vi "Basic_SetupBoard.vi"() -> ()   [LabVIEW 2020]
uses:
  controls/basic_tx_states.ctl
  AIM664LV.lvlib
panel:
  in  "Explicit libInit (T)":bool=TRUE
  out "BSP Version Out":T1
  out "Board Control Out":T2 {"SharedMemFree" format="%x"; "GlobalMemFree" format="%x"; "ExpertMode" items=["FDX_EXPERT_MODE", "FDX_DISA_GHOST"]; "PortGoodLink" items=["FDX_NO_LINK", "FDX_GOOD_LINK"]; "PortSpeed" items=["FDX_100MBIT", "FDX_10MBIT", "FDX_AUTO_100MBIT", "FDX_AUTO_10MBIT", "FDX_AUTO_ERROR", "FDX_1000MBIT"]; "PortConfig" items=["FDX_SINGLE", "FDX_REDUNDANT"]}
  in  "ExpertMode":u32(ring) items=["FDX_EXPERT_MODE", "FDX_DISA_GHOST"]
  in  "PortSpeedIn":u32(ring) items=["FDX_100MBIT"=0, "FDX_10MBIT"=1, "FDX_AUTO_100MBIT"=2, "FDX_AUTO_10MBIT"=3, "FDX_1000MBIT"=5]
  in  "PortConfigIn":u32(ring) items=["FDX_SINGLE", "FDX_REDUNDANT"]
  in  "Control":u32(ring) items=["FDX_READ", "FDX_WRITE"]
  out "error out":errorcluster
  out "ServerResourceInfo":T3(array[cluster]) {"ResourceType" items=["RESOURCETYPE_BOARD"=0, "RESOURCETYPE_PORT"=1, "RESOURCETYPE_ALL"=20]}
  out "NuOfServers":u32
  # "#define FDX_100MBIT        0\n#define FDX_10MBIT         1\n#define FDX_AUTO_100MBIT   2\n#define FDX_AUTO_10MBIT    3\n#define FDX_AUTO_ERROR     4\n#define FDX_1000MBIT       5"
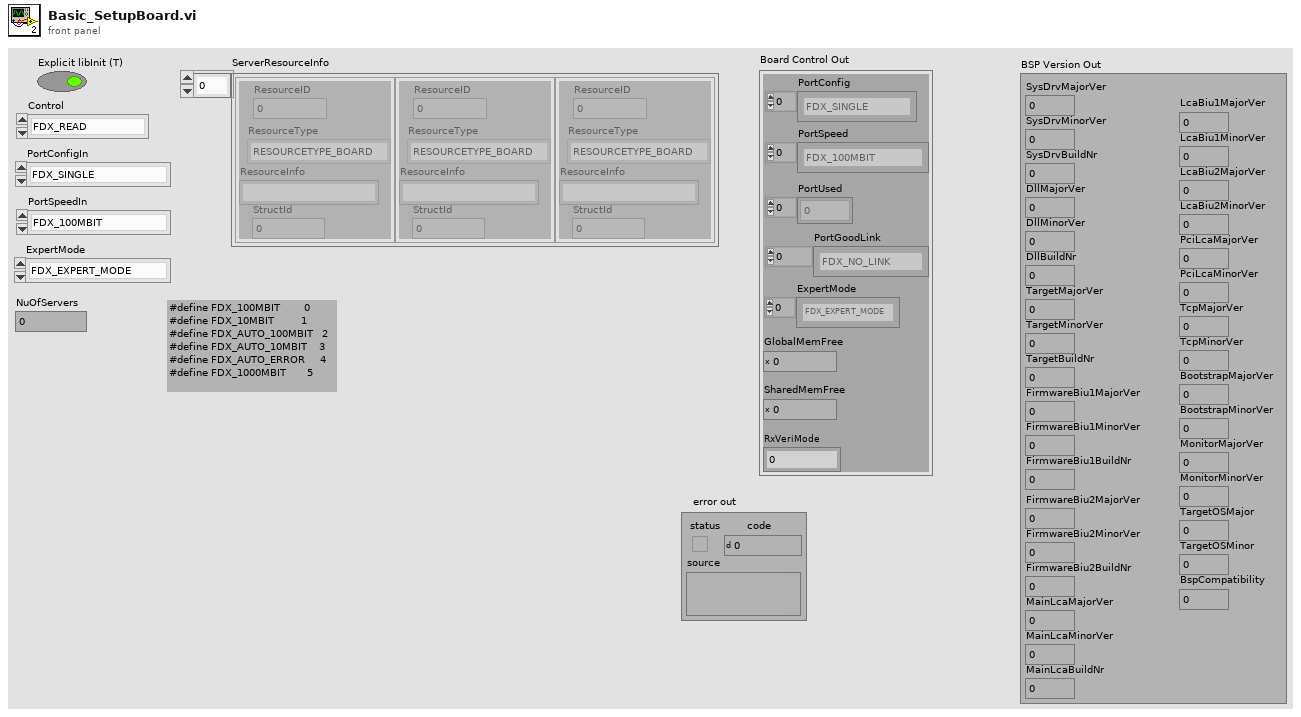
[diagram p1: front panel]
types:
  T1 = cluster{"SysDrvMajorVer":u32, "SysDrvMinorVer":u32, "SysDrvBuildNr":u32, "DllMajorVer":u32, "DllMinorVer":u32, "DllBuildNr":u32, "TargetMajorVer":u32, "TargetMinorVer":u32, "TargetBuildNr":u32, "FirmwareBiu1MajorVer":u32, "FirmwareBiu1MinorVer":u32, "FirmwareBiu1BuildNr":u32, "FirmwareBiu2MajorVer":u32, "FirmwareBiu2MinorVer":u32, "FirmwareBiu2BuildNr":u32, "MainLcaMajorVer":u32, "MainLcaMinorVer":u32, "MainLcaBuildNr":u32, "LcaBiu1MajorVer":u32, "LcaBiu1MinorVer":u32, "LcaBiu2MajorVer":u32, "LcaBiu2MinorVer":u32, "PciLcaMajorVer":u32, "PciLcaMinorVer":u32, "TcpMajorVer":u32, "TcpMinorVer":u32, "BootstrapMajorVer":u32, "BootstrapMinorVer":u32, "MonitorMajorVer":u32, "MonitorMinorVer":u32, "TargetOSMajor":u32, "TargetOSMinor":u32, "BspCompatibility":u32}
  T2 = cluster{"PortConfig":u32[], "PortSpeed":u32[], "PortUsed":u32[], "PortGoodLink":u32[], "ExpertMode":u32[], "GlobalMemFree":u32, "SharedMemFree":u32, "RxVeriMode":u32}
  T3 = cluster{"ResourceID":u32, "ResourceType":u32, "ResourceInfo":string, "StructId":u32}[]
  T4 = typedef "basic_tx_states.ctl" = enum16{"InitAndLogin", "BoardSetup", "TxModeSetup", "TxTransmissionControl", "GenerateTraffic", "LogoutAndRelease"}
  T5 = cluster{"Control":u32, "Port1ConfigIn":u32, "Port2ConfigIn":u32, "Port3ConfigIn":u32, "Port4ConfigIn":u32, "Port1SpeedIn":u32, "Port2SpeedIn":u32, "Port3SpeedIn":u32, "Port4SpeedIn":u32, "Expert1Mode":u32, "Expert2Mode":u32, "Expert3Mode":u32, "Expert4Mode":u32, "RxVeriModeIn":u32, "RxVeriData1":u32, "RxVeriData2":u32, "RxVeriData3":u32, "RxVeriData4":u32, "RxVeriData5":u32, "RxVeriData6":u32, "RxVeriData7":u32, "RxVeriData8":u32, "RxVeriMask1":u32, "RxVeriMask2":u32, "RxVeriMask3":u32, "RxVeriMask4":u32, "RxVeriMask5":u32, "RxVeriMask6":u32, "RxVeriMask7":u32, "RxVeriMask8":u32}
  T6 = typedef "AIM664LV.lvlib/port_configuration.ctl" = u32
  T7 = typedef "AIM664LV.lvlib/port_speed.ctl" = u32
  T8 = typedef "AIM664LV.lvlib/port_condition.ctl" = u32
  T9 = typedef "AIM664LV.lvlib/expert_mode.ctl" = u32
  T10 = cluster{"PortConfig":T6[], "PortSpeed":T7[], "PortUsed":u32[], "PortGoodLink":T8[], "ExpertMode":T9[], "GlobalMemFree":u32, "SharedMemFree":u32, "RxVeriMode":u32}
  T11 = cluster{"SrvName":string, "ResourceID":u32, "ResourceType":u32}
  T12 = cluster{"SrvName":string, "ClHostName":string, "ClUser":string, "ClApplication":string, "ClApplicationVersion":string, "ResourceID":u32, "Privileges":u32}
  T13 = cluster{"ResourceID":u32, "ResourceType":u32, "ResourceInfo":string, "StructId":u32}
  T14 = cluster{"BoardName":string, "BoardSerialNo":u32, "BoardNumOf\nEthernetPorts":u32, "BoardClients":u32, "BoardGlobal\nMemSize":u32, "BoardShared\nMemSize":u32, "BoardStructId":u32, "PortName":string, "PortMode":u32, "PortNo":u32, "PortBoard\nResourceID":u32, "PortStructId":u32}
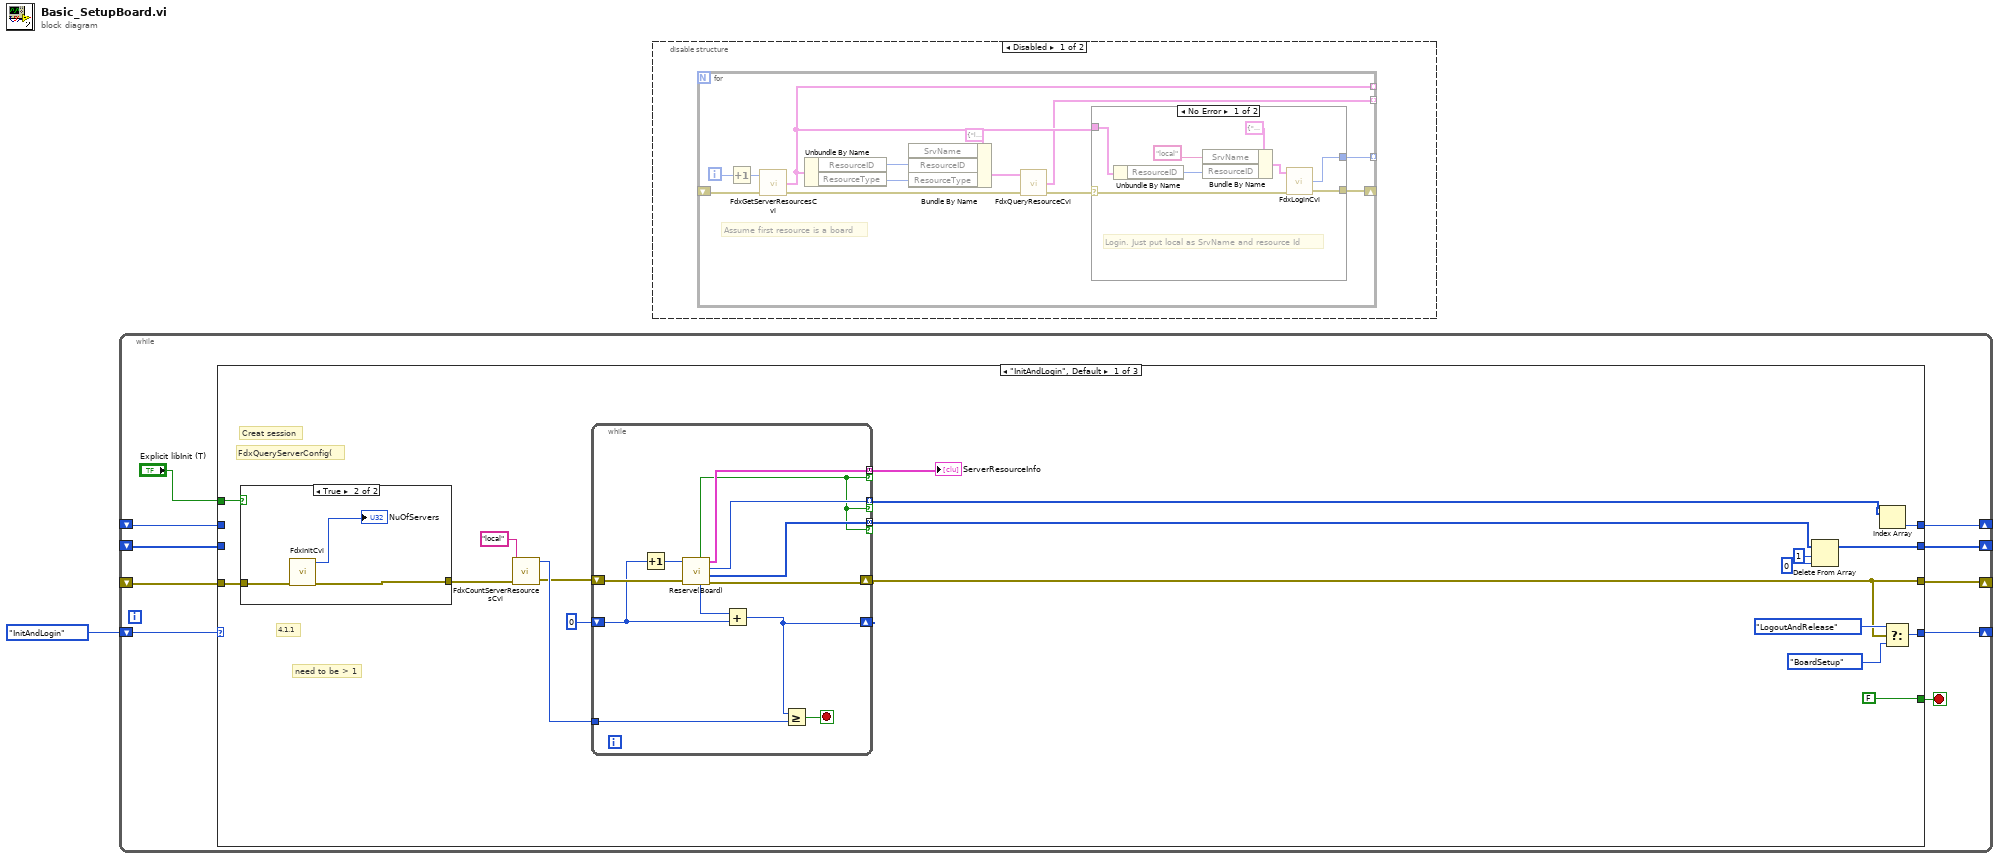
[diagram p0: block diagram]
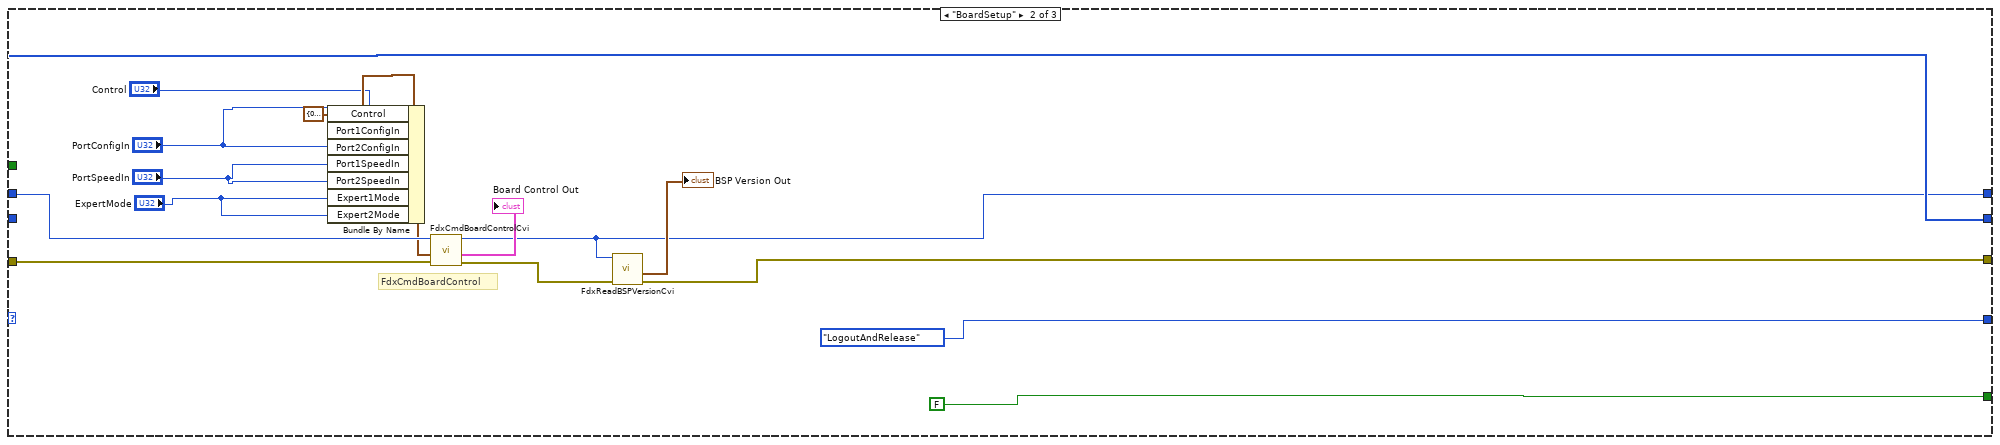
[diagram p5: hidden frame]
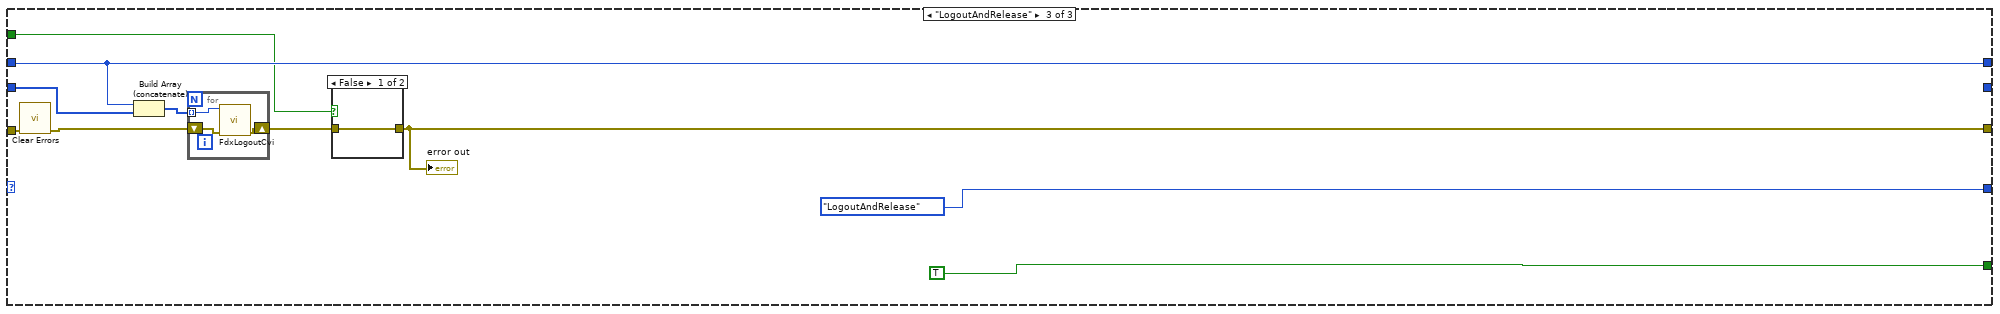
[diagram p6: hidden frame]
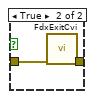
[diagram p7: hidden frame]
diagram:
  n1 = while {
    shift-right: [w8] -> _
    shift-left: basic_tx_states."InitAndLogin" -> [w10]
    shift-right: [w9] -> _
    shift-left: _ -> [w7]
    shift-right: [w6] -> _
    shift-left: _ -> [w4]
    shift-right: [w5] -> _
    shift-left: _ -> [w3]
    stop <- w11 stop-if-true
    n2 = case shown="\"InitAndLogin\", Default" w10 {
      tunnel: [FALSE FALSE TRUE] -> w11
      tunnel: [w17 w49 w70] -> w9
      tunnel: [w26 basic_tx_states."LogoutAndRelease" basic_tx_states."LogoutAndRelease"] -> w8
      tunnel: w7 -> [w25 w62 w69]
      tunnel: [w13 w47 w66] -> w6
      tunnel: [w22 w55 _] -> w5
      tunnel: w4 -> [_ w61 w66]
      tunnel: w3 -> [_ w55 w64]
      tunnel: "Explicit libInit (T)" -> [w12 _ w63]
      frame "InitAndLogin", Default {
        # "FdxQueryServerConfig("
        # "need to be > 1"
        # "Creat session"
        # "4.1.1"
        n3 = case shown="True" w12 {
          tunnel: [w31 w33] -> w29
          tunnel: w25 -> [w31 w32]
          frame False {
          }
          frame True {
            n4 = call "FdxInitCvi.vi"("error in"=w32) -> ("error out"=w33:errorcluster, "Number of Servers"=→"NuOfServers":u32)  [unwired: 9 in]
          }
        }
        n5 = call "FdxCountServerResourcesCvi.vi"("error in"=w29, "SrvName (local)"="local" ("SrvName")) -> ("error out"=w19:errorcluster, "Number of Resources"=w20:u32)  [unwired: 8 in]
        n6 = while {
          tunnel: w20 -> [w46]
          shift-right: [w39] -> w17
          shift-left: w19 -> [w44]
          shift-right: [w40] -> _
          shift-left: 0 -> [w41]
          tunnel: [w38] -> w16 mode=concatenating if=w35
          tunnel: [w37] -> w15 mode=indexing if=w35
          tunnel: [w36] -> w14 mode=concatenating if=w35
          stop <- w45 stop-if-true
          n7 = Increment(x=w41) -> (x+1=w43:i32)
          n8 = call "Reserve(Board).vi"("error in"=w44, "ServerRElement"=w43) -> ("error out"=w39:errorcluster, "PortHandles"=w36:u32[], "BoardHandle"=w37:u32, "Resources"=w38:T3, "elements found"=w42:i32, "found"=w35:bool)  [unwired: 4 in]
          n9 = Add(x=w42, y=w41) -> (x+y=w40:i32)
          n10 = Greater Or Equal?(x=w40, y=w46) -> (x >= y?=w45:bool)
        }
        "ServerResourceInfo" <- w16
        n11 = Delete From Array(array=w14, length=1, index=0 ("length")) -> (array with subset deleted=w22:u32[])  [unwired: 1 out]
        n12 = Index Array(array=w15) -> (element=w13:u32)  [unwired: 1 in]
        n13 = Select(t=basic_tx_states."LogoutAndRelease", s=w17, f=basic_tx_states."BoardSetup") -> (s? t:f=w26:T4)
      }
      frame "BoardSetup" {
        # "FdxCmdBoardControl"
        n14 = Bundle By Name(cluster=T5 {"Control"=0, "Port1ConfigIn"=0, "Port2ConfigIn"=0, "Port3ConfigIn"=0, "Port4ConfigIn"=0, "Port1SpeedIn"=0, "Port2SpeedIn"=0, "Port3SpeedIn"=0, "Port4SpeedIn"=0, "Expert1Mode"=0, "Expert2Mode"=0, "Expert3Mode"=0, "Expert4Mode"=0, "RxVeriModeIn"=0, "RxVeriData1"=0, "RxVeriData2"=0, "RxVeriData3"=0, "RxVeriData4"=0, "RxVeriData5"=0, "RxVeriData6"=0, "RxVeriData7"=0, "RxVeriData8"=0, "RxVeriMask1"=0, "RxVeriMask2"=0, "RxVeriMask3"=0, "RxVeriMask4"=0, "RxVeriMask5"=0, "RxVeriMask6"=0, "RxVeriMask7"=0, "RxVeriMask8"=0} ("BoardControlIn"), "Control"="Control", "Port1ConfigIn"="PortConfigIn", "Port2ConfigIn"="PortConfigIn", "Port1SpeedIn"="PortSpeedIn", "Port2SpeedIn"="PortSpeedIn", "Expert1Mode"="ExpertMode", "Expert2Mode"="ExpertMode") -> (w59:T5)
        n15 = call "FdxCmdBoardControlCvi.vi"("error in"=w62, "BoardControlIn (read)"=w59, "InstrumentHandle_board in"=w61) -> ("error out"=w50:errorcluster, "Board Control Out"=→"Board Control Out":T10, "InstrumentHandle_board out"=w47:u32)  [unwired: 6 in]
        n16 = call "FdxReadBSPVersionCvi.vi"("error in"=w50, "InstrumentHandle_board in"=w47) -> ("error out"=w49:errorcluster, "BSP Version Out"=→"BSP Version Out":T1)  [unwired: 7 in, 1 out]
      }
      frame "LogoutAndRelease" {
        n17 = call <vilib>:"Clear Errors.vi"("error in (no error)"=w69) -> ("error out"=w68:errorcluster)  [unwired: 5 in, 1 out]
        n18 = Build Array (concatenate)(w66, w64) -> (w65:u32[])
        n19 = for {
          shift-right: [w77] -> w67
          shift-left: w68 -> [w78]
          tunnel: w65 -> [w76] mode=indexing
          n20 = call "FdxLogoutCvi.vi"("error in"=w78, "InstrumentHandle"=w76) -> ("error out"=w77:errorcluster)  [unwired: 9 in]
        }
        n21 = case shown="False" w63 {
          tunnel: [w73 w75] -> w70
          tunnel: w67 -> [w73 w74]
          frame False {
          }
          frame True {
            n22 = call "FdxExitCvi.vi"("error in"=w74) -> ("error out"=w75:errorcluster)  [unwired: 10 in]
          }
        }
        "error out" <- w70
      }
    }
  }
  n23 = disable-structure shown="Disabled" {
    frame Disabled {
      n24 = for {
        shift-right: [w88] -> _
        shift-left: _ -> [w91]
        tunnel: [w82] -> _ mode=indexing
        tunnel: [w87] -> _ mode=indexing
        tunnel: [w79] -> _ mode=indexing
        i -> [w89]
        # "Assume first resource is a board"
        n25 = Increment(x=w89) -> (x+1=w90:i32)
        n26 = call "FdxGetServerResourcesCvi.vi"("error in (no error)"=w91, "ServerRElement"=w90) -> ("error out"=w86:errorcluster, "ServerResourceInfo"=w82:T13)  [unwired: 1 in, 1 out]
        n27 = Unbundle By Name(w82) -> ("ResourceID"=w81:u32, "ResourceType"=w80:u32)
        n28 = Bundle By Name(cluster=T11 {"SrvName"="local", "ResourceID"=0, "ResourceType"=0} ("QueryResource"), "ResourceID"=w81, "ResourceType"=w80) -> (w84:T11)  [unwired: 1 in]
        n29 = call "FdxQueryResourceCvi.vi"("error in (no error)"=w86, "QueryResource"=w84) -> ("error out"=w83:errorcluster, "ResourceInfo"=w79:T14)  [unwired: 1 in, 1 out]
        n30 = case shown="No Error" w83 {
          selector: w83 -> [w94 w100]
          tunnel: w82 -> [w99 _]
          tunnel: [w93 w100] -> w88
          tunnel: [w92 _] -> w87
          frame No Error {
            # "Login. Just put local as SrvName and resource Id"
            n31 = Unbundle By Name(w99) -> ("ResourceID"=w96:u32)
            n32 = Bundle By Name(cluster=T12 {"SrvName"="", "ClHostName"="", "ClUser"="", "ClApplication"="", "ClApplicationVersion"="", "ResourceID"=0, "Privileges"=4294967295} ("ClientInfo"), "SrvName"="local", "ResourceID"=w96) -> (w95:T12)
            n33 = call "FdxLoginCvi.vi"("error in (no error)"=w94, "ClientInfo"=w95) -> ("error out"=w93:errorcluster, "InstrumentHandle"=w92:u32)  [unwired: 1 in, 1 out]
          }
          frame Error {
          }
        }
      }
    }
    frame Enabled {
    }
  }
